vi "Scan_normailze(SubVI).vi"(8 "error in (no error)":errorcluster, 9 "Channel index (0-23)":u8=14, 10 "Normalization":bool=TRUE, 11 "Application in":refnum<vi>) -> (0 "error out":errorcluster, 2 "Array":dbl[][](array[numeric]), 3 "Application out":refnum<vi>)   [LabVIEW 2014]
uses:
  <userlib>/Nanonis Prog Interface V5/Nanonis Prog Interface.lvlib
panel:
  out "Channel name":string
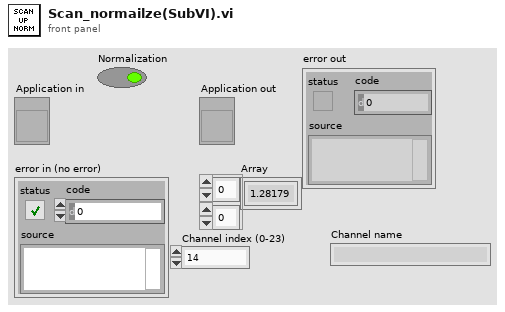
[diagram p1: front panel]
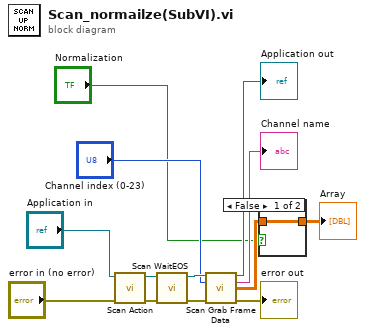
[diagram p0: block diagram]
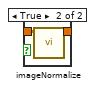
[diagram p2: hidden frame]
diagram:
  n1 = call <userlib>:"Scan Action.vi"("error in (no error)"="error in (no error)", "Application ref in"="Application in") -> ("error out"=w5:errorcluster, "Application ref out"=w6:refnum<vi>)  [unwired: 7 in]
  n2 = call <userlib>:"Scan WaitEOS.vi"("error in (no error)"=w5, "Application ref in"=w6) -> ("error out"=w7:errorcluster, "Application ref out"=w8:refnum<vi>)  [unwired: 5 in, 2 out]
  n3 = call <userlib>:"Scan Grab Frame Data.vi"("Application ref in"=w8, "Channel index (0-23)"="Channel index (0-23)", "error in (no error)"=w7) -> ("Application ref out"=→"Application out":refnum<vi>, "Channel name"=→"Channel name":string, "Scan frame data"=w12:sgl[][], "error out"=→"error out":errorcluster)  [unwired: 8 in, 1 out]
  n4 = case shown="False" "Normalization" {
    tunnel: [w14 w16] -> w13
    tunnel: w12 -> [w14 w15]
    frame False {
    }
    frame True {
      n5 = call "imageNormalize.vi"("Data"=w15) -> ("Array"=w16:dbl[][])  [unwired: 10 in]
    }
  }
  "Array" <- w13
